vi "MaxsGettoArcadeDrive.vi"(10 "Driver X In":dbl, 11 "Driver Y In":dbl) -> (2 "Right Out":dbl, 3 "Left Out":dbl)   [LabVIEW 2012]
uses:
  Max'sToolKit/ConvertVoltageToPercentVbs.vi
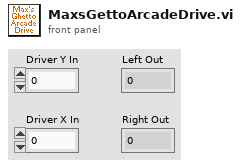
[diagram p1: front panel]
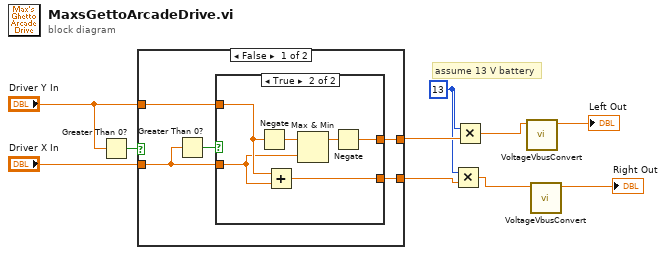
[diagram p0: block diagram]
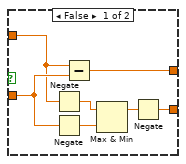
[diagram p2: hidden frame]
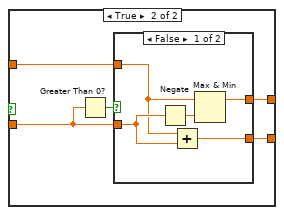
[diagram p3: hidden frame]
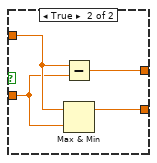
[diagram p4: hidden frame]
diagram:
  w3 = 13
  # "assume 13 V battery"
  n1 = Greater Than 0?(x="Driver Y In") -> (x > 0?=w10:bool)
  n2 = case shown="False" w10 {
    tunnel: "Driver X In" -> [w14 w32]
    tunnel: "Driver Y In" -> [w13 w31]
    tunnel: [w12 w30] -> w4
    tunnel: [w11 w29] -> w5
    frame False {
      n3 = Greater Than 0?(x=w14) -> (x > 0?=w15:bool)
      n4 = case shown="True" w15 {
        tunnel: w14 -> [w22 w24]
        tunnel: w13 -> [w20 w25]
        tunnel: [w16 w26] -> w12
        tunnel: [w17 w23] -> w11
        frame False {
          n5 = Negate(x=w20) -> (-x=w21:dbl)
          n6 = Negate(x=w22) -> (-x=w19:dbl)
          n7 = Subtract(x=w20, y=w22) -> (x-y=w16:dbl)
          n8 = Max & Min(x=w21, y=w19) -> (max(x,y)=w18:dbl)  [unwired: 1 out]
          n9 = Negate(x=w18) -> (-x=w17:dbl)
        }
        frame True {
          n10 = Negate(x=w25) -> (-x=w28:dbl)
          n11 = Add(x=w25, y=w24) -> (x+y=w23:dbl)
          n12 = Max & Min(x=w28, y=w24) -> (max(x,y)=w27:dbl)  [unwired: 1 out]
          n13 = Negate(x=w27) -> (-x=w26:dbl)
        }
      }
    }
    frame True {
      n14 = Greater Than 0?(x=w32) -> (x > 0?=w33:bool)
      n15 = case shown="False" w33 {
        tunnel: w32 -> [w38 w40]
        tunnel: w31 -> [w35 w41]
        tunnel: [w36 w39] -> w30
        tunnel: [w34 w42] -> w29
        frame False {
          n16 = Negate(x=w38) -> (-x=w37:dbl)
          n17 = Add(x=w35, y=w38) -> (x+y=w34:dbl)
          n18 = Max & Min(x=w35, y=w37) -> (max(x,y)=w36:dbl)  [unwired: 1 out]
        }
        frame True {
          n19 = Subtract(x=w41, y=w40) -> (x-y=w39:dbl)
          n20 = Max & Min(x=w41, y=w40) -> (max(x,y)=w42:dbl)  [unwired: 1 out]
        }
      }
    }
  }
  n21 = Multiply(x=w3, y=w5) -> (x*y=w2:dbl)
  n22 = Multiply(x=w3, y=w4) -> (x*y=w1:dbl)
  n23 = call-poly "VoltageVbusConvert.vi"("Voltage"=w1) -> ("Vbus"=→"Left Out":dbl)  [unwired: 10 in]
  n24 = call-poly "VoltageVbusConvert.vi"("Voltage"=w2) -> ("Vbus"=→"Right Out":dbl)  [unwired: 10 in]
